vi "Execute SQL.vi"(8 "error in (no error)":errorcluster, 9 "[disabled] return type (string)":string, 10 "sql (string)":string="SELECT * FROM employees;", 11 "database in":path=path "C:/labview/sqlite_dbManager/test/chinook.db") -> (0 "error out":errorcluster, 2 "Query Result":string[][](array[string]))   [LabVIEW 2020, in "sqlite3.lvlib"]
uses:
  sqlite3.lvlib
  sqlite/subvi/Error Converter (ErrCode or Status).vi
  sqlite/VIs/column text.vi
  sqlite/VIs/column bytes.vi
  sqlite/VIs/column blob.vi
  utilities/MoveBlock.vi
  sqlite/VIs/column type.vi
  sqlite/VIs/errstr.vi
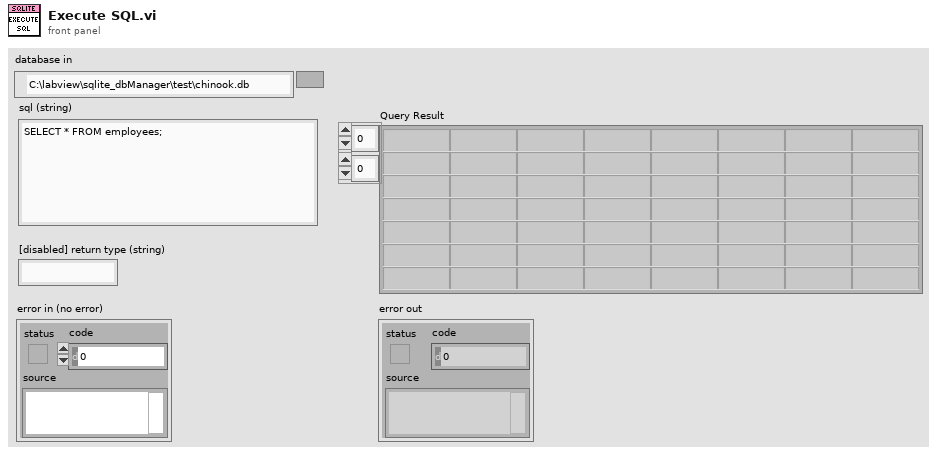
[diagram p1: front panel]
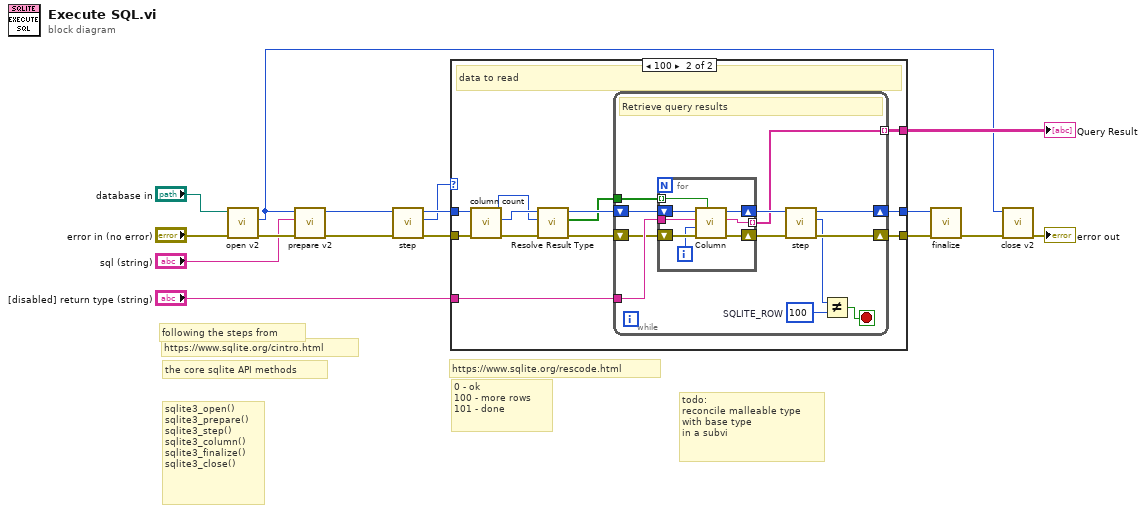
[diagram p0: block diagram]
diagram:
  # "todo:\nreconcile malleable type\nwith base type\nin a subvi"
  # "the core sqlite API methods"
  # "following the steps from"
  # "0 - ok\n100 - more rows\n101 - done"
  # "https://www.sqlite.org/rescode.html"
  # "sqlite3_open()\nsqlite3_prepare()\nsqlite3_step()\nsqlite3_column()\nsqlite3_finalize()\nsqlite3_close()"
  # "https://www.sqlite.org/cintro.html"
  n1 = call "open v2.vi"("error in (no error)"="error in (no error)", "filename"="database in") -> ("error out"=w13:errorcluster, "ppDb out"=w2:u64)  [unwired: 8 in]
  n2 = call "prepare v2.vi"("error in (no error)"=w13, "zSql"="sql (string)", "db"=w2) -> ("error out"=w11:errorcluster, "ppStmt out"=w1:u64)  [unwired: 6 in, 1 out]
  n3 = call "step.vi"("error in (no error)"=w11, "para0"=w1) -> ("error out"=w9:errorcluster, "sqlite3_step"=w8:i32, "para0 out"=w10:u64)  [unwired: 7 in]
  n4 = case shown="100" w8 {
    tunnel: w10 -> [w18 w30]
    tunnel: w9 -> [w17 w29]
    tunnel: [w17 w27] -> w7
    tunnel: [w18 w28] -> w6
    tunnel: "[disabled] return type (string)" -> [_ w26]
    tunnel: [_ w25] -> w3
    frame 0, 101, Default {
      # "no data"
    }
    frame 100 {
      # "data to read"
      n5 = call "column count.vi"("error in (no error)"=w29, "pStmt"=w30) -> ("error out"=w24:errorcluster, "#cols"=w22:i32, "pStmt out"=w21:u64)  [unwired: 7 in]
      n6 = call "Resolve Result Type.vi"("error in (no error)"=w24, "pStmt in"=w21, "#cols"=w22) -> ("error out"=w23:errorcluster, "blob?"=w19:bool[], "pStmt out"=w20:u64)  [unwired: 5 in, 1 out]
      n7 = while {
        shift-right: [w42] -> w28
        shift-left: w20 -> [w34]
        shift-right: [w41] -> w27
        shift-left: w23 -> [w33]
        tunnel: w26 -> [w35]
        tunnel: [w36] -> w25 mode=indexing
        tunnel: w19 -> [w31]
        stop <- w38 stop-if-true
        w39 = 100  # SQLITE_ROW
        # "Retrieve query results"
        n8 = for {
          shift-right: [w50] -> w37
          shift-left: w34 -> [w44]
          tunnel: [w49] -> w36 mode=indexing
          tunnel: w35 -> [w45]
          shift-right: [w47] -> w32
          shift-left: w33 -> [w48]
          tunnel: w31 -> [w43] mode=indexing
          i -> [w46]
          n9 = call "Column.vi"("Blob?"=w43, "error in (no error)"=w48, "iCol"=w46, "query return type"=w45, "para0"=w44) -> ("error out"=w47:errorcluster, "function return"=w49:string, "para0 out"=w50:u64)  [unwired: 4 in]
        }
        n10 = call "step.vi"("error in (no error)"=w32, "para0"=w37) -> ("error out"=w41:errorcluster, "sqlite3_step"=w40:i32, "para0 out"=w42:u64)  [unwired: 7 in]
        n11 = Not Equal?(x=w40, y=w39) -> (x != y?=w38:bool)
      }
    }
  }
  "Query Result" <- w3
  n12 = call "finalize.vi"("error in (no error)"=w7, "pStmt"=w6) -> ("error out"=w5:errorcluster)  [unwired: 9 in]
  n13 = call "close v2.vi"("error in (no error)"=w5, "para0"=w2) -> ("error out"=→"error out":errorcluster)  [unwired: 9 in]
